vi "eng-error-handler.vi"(8 "error in":errorcluster, 10 "Numeric":dbl) -> (0 "error out":errorcluster, 2 "delta t":dbl)   [LabVIEW 2024]
uses:
  <vilib>/Utility/error.llb/DialogType.ctl
  controls/typeEngErrorCodes.ctl
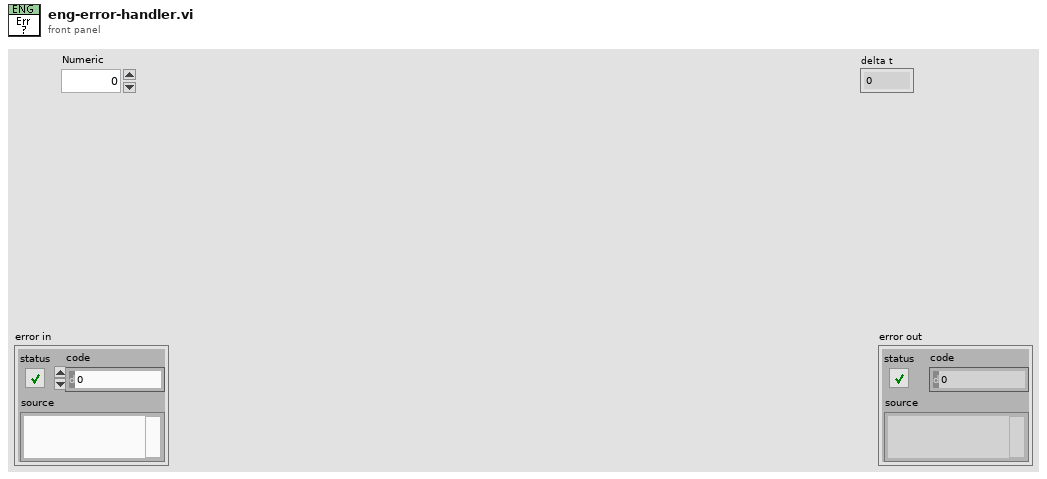
[diagram p1: front panel]
types:
  T1 = typedef "typeEngErrorCodes.ctl" = u16
  T2 = typedef "DialogType.ctl" = u16
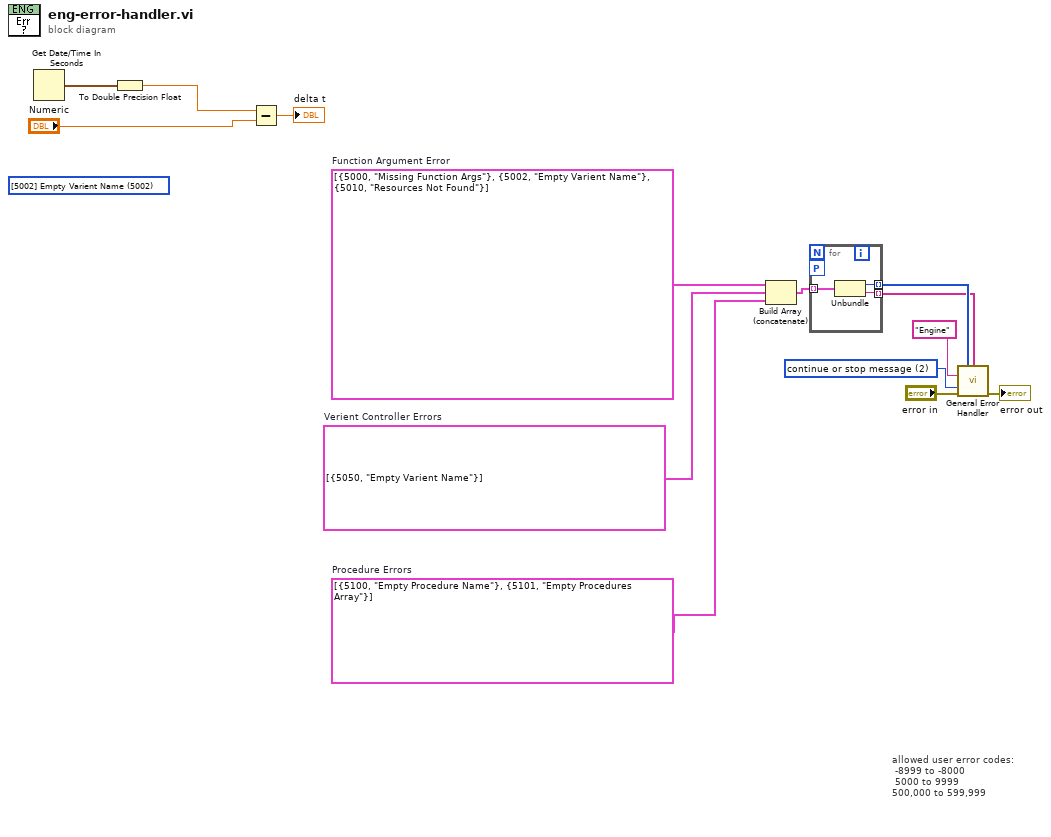
[diagram p0: block diagram]
diagram:
  w6 = cluster{i32, string}[] [{5100, "Empty Procedure Name"}, {5101, "Empty Procedures Array"}]  # Procedure Errors
  w7 = cluster{i32, string}[] [{5050, "Empty Varient Name"}]  # Verient Controller Errors
  w11 = cluster{i32, string}[] [{5000, "Missing Function Args"}, {5002, "Empty Varient Name"}, {5010, "Resources Not Found"}]  # Function Argument Error
  (unwired) T1 5002 items=["[5000] Missing Function Arguments"=5000, "[5001] Incorrect Function Arguments"=5001, "[5002] Empty Varient Name"=5002, "[5010] Not Found"=5010] ("Ring")
  w14 = T2 2 items=["no dialog", "OK message", "continue or stop message", "OK message + warnings", "continue/stop + warnings"] ("type of dialog (OK msg:1)")
  # "allowed user error codes:\n -8999 to -8000\n 5000 to 9999\n500,000 to 599,999"
  n1 = Get Date/Time In Seconds() -> (seconds since 1Jan1904=w2:timestamp)
  n2 = To Double Precision Float(number=w2) -> (double precision float=w1:dbl)
  n3 = Subtract(x=w1, y="Numeric") -> (x-y=→"delta t":dbl)
  n4 = Build Array (concatenate)(w11, w7, w6) -> (w8:cluster{i32, string}[])
  n5 = for {
    tunnel: w8 -> [w17] mode=indexing
    tunnel: [w16] -> w9 mode=indexing
    tunnel: [w15] -> w10 mode=indexing
    workers-P: _ -> [_]
    n6 = Unbundle(w17) -> (w15:i32, w16:string)
  }
  n7 = call <vilib>:"General Error Handler.vi"("[user-defined codes]"=w10, "[user-defined descriptions]"=w9, "[error source] (\" \")"="Engine" ("[error source] (\" \")"), "type of dialog (OK msg:1)"=w14, "error in (no error)"="error in") -> ("error out"=→"error out":errorcluster)  [unwired: 6 in, 4 out]
